vi "Get SMO Serial Number.vi"(8 "error in (no error)":errorcluster, 11 "Inst.RP100 in":refnum<class "Inst.RP100.lvclass">) -> (0 "error out":errorcluster, 2 "Serial Number":string, 3 "Inst.RP100 out":refnum<class "Inst.RP100.lvclass">)   [LabVIEW 2019, in "Inst.RP100.lvlib" / "Inst.RP100.lvclass"]
doc: "Override this VI to return the serial number of your Instrument"
uses:
  Inst.RP100.lvclass
  Inst.RP100.lvclass/Inst.RP100.ctl
  RP100/RP100.lvlib
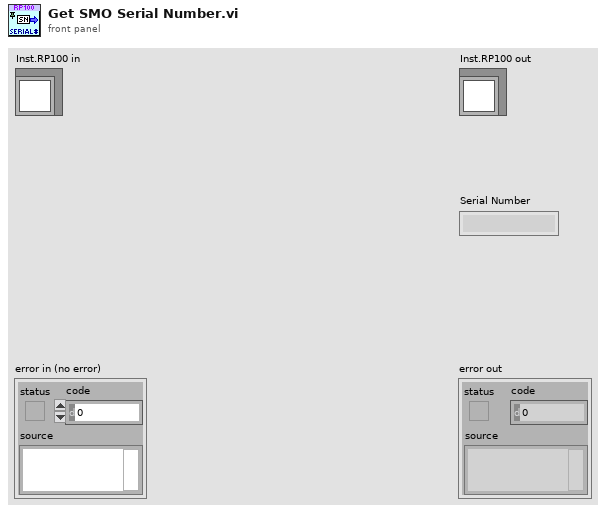
[diagram p1: front panel]
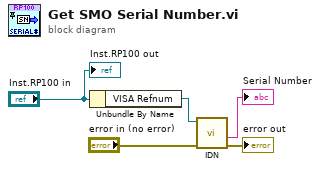
[diagram p0: block diagram]
diagram:
  n1 = Unbundle By Name("Inst.RP100 in") -> ("VISA Refnum"=w1:refnum<visa-resource-name>)
  n2 = call "IDN.vi"("error in (no error)"="error in (no error)", "VISA resource name"=w1) -> ("error out"=→"error out":errorcluster, "Serial Number"=→"Serial Number":string)  [unwired: 4 in, 4 out]
  "Inst.RP100 out" <- "Inst.RP100 in"
